vi "Flatten Cluster To CfgTable.vi"(8 "error in (no error)":errorcluster, 11 "Cluster Configuration Typedef":variant) -> (0 "error out":errorcluster, 3 "CfgTable Row":string[](array[string]))   [LabVIEW 2017, in "ClusterCfgTable.lvlib"]
doc: "Converts a cluster into a two-dimensional configuration table from the cluster's own type information, without data names. It is the simple entry point to Flatten Cluster To CfgTable(with DataName).vi."
uses:
  ClusterCfgTable.lvlib
panel:
  in  "ConfigStrings Typedef":string[](array[string])
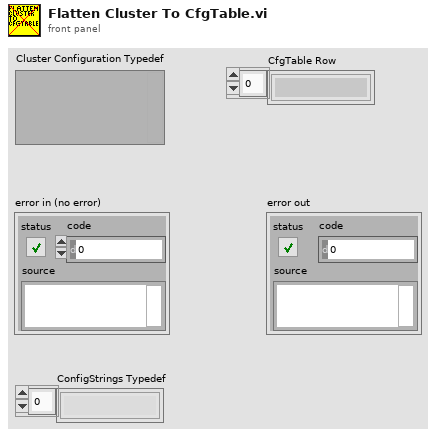
[diagram p1: front panel]
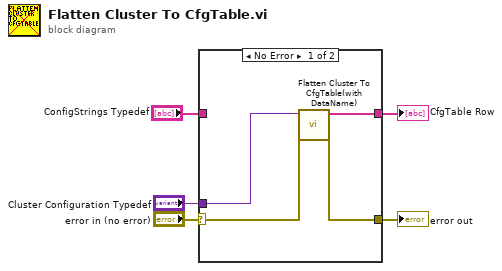
[diagram p0: block diagram]
diagram:
  n1 = case shown="No Error" "error in (no error)" {
    selector: "error in (no error)" -> [w8 w11]
    tunnel: [w9 w11] -> w5
    tunnel: "Cluster Configuration Typedef" -> [w7 _]
    tunnel: [w6 w10] -> w2
    tunnel: "ConfigStrings Typedef" -> [_ w10]
    frame No Error {
      n2 = call "Flatten Cluster To CfgTable(with DataName).vi"("error in (no error)"=w8, "Cluster Configuration Typedef"=w7) -> ("error out"=w9:errorcluster, "CfgTable Row"=w6:string[])  [unwired: 7 in, 1 out]
    }
    frame Error {
    }
  }
  "CfgTable Row" <- w2
  "error out" <- w5
